vi "Add Drawable.vi"(10 "Drawable":refnum<class "Drawable.lvclass">, 11 "Game Board in":refnum<class "Game Board.lvclass">) -> (3 "Game Board out":refnum<class "Game Board.lvclass">)   [LabVIEW 2020, in "Game Board.lvclass"]
uses:
  Game Board.lvclass
  Drawable/Drawable.lvclass
  Game Board.lvclass/Game Board.ctl
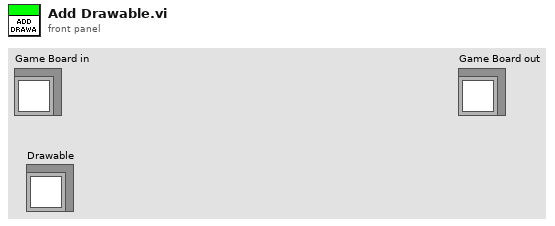
[diagram p1: front panel]
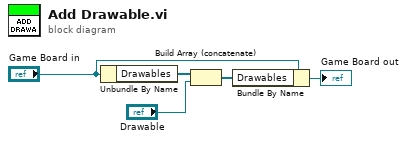
[diagram p0: block diagram]
diagram:
  n1 = Unbundle By Name("Game Board in") -> ("Drawables"=w3:refnum<class "Drawable.lvclass">[])
  n2 = Build Array (concatenate)(w3, "Drawable") -> (w1:refnum<class "Drawable.lvclass">[])
  n3 = Bundle By Name(cluster="Game Board in", "Drawables"=w1) -> (→"Game Board out":refnum<class "Game Board.lvclass">)
